vi "Set PressureDisplay Setup.vi"(8 "error in (no error)":errorcluster, 10 "PressureDisplay Setup":T1[](array[typedef]) {"Threshold" format="%#.1e"}, 11 "VacuumLines Configuration in":refnum<class "VacuumLines Configuration.lvclass">) -> (0 "error out":errorcluster, 3 "VacuumLines Configuration out":refnum<class "VacuumLines Configuration.lvclass">)   [LabVIEW 2016, in "Hardware.lvlib" / "VacuumLine.lvlib" / "VacuumLines Configuration.lvclass"]
uses:
  <userlib>/Common Components/Hardware/Abstract System/VacuumLine/VacuumLines Configuration/VacuumLines Configuration.lvclass
  <userlib>/Common Components/Hardware/Abstract System/VacuumLine/VacuumLines/Gauge Param.ctl
  <userlib>/Common Components/Hardware/Abstract System/VacuumLine/VacuumLines Configuration/VacuumLines Configuration.lvclass/VacuumLines Configuration.ctl
  <userlib>/Common Components/Hardware/Abstract System/VacuumLine/VacuumLines/VacuumLines.lvclass/VacuumLines.ctl
  <userlib>/Common Components/Hardware/Abstract System/VacuumLine/VacuumLines/VacuumLines.lvclass
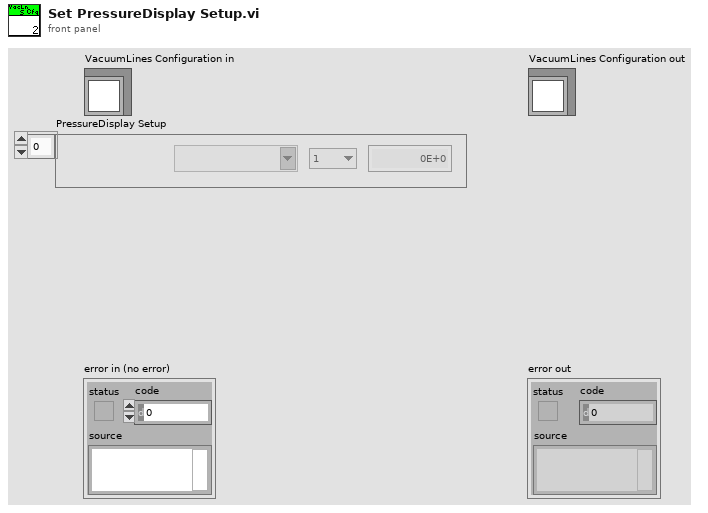
[diagram p1: front panel]
types:
  T1 = typedef "Hardware.lvlib/VacuumLine.lvlib/VacuumLines.lvclass/Gauge Param.ctl" = cluster{"label":string, "Gauge Controller":string, "Channel":enum16{"1", "2", "3", "4", "5", "6", "7", "8"}, "Threshold":dbl}
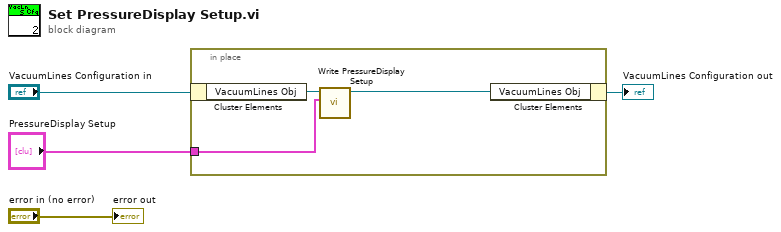
[diagram p0: block diagram]
diagram:
  n1 = in-place {
    in-place-border: "PressureDisplay Setup" -> [w5]
    n2 = in-place-cluster #1("VacuumLines Configuration in") -> ("VacuumLines Obj"=w7:refnum<class "VacuumLines.lvclass">)
    n3 = call <userlib>:"Write PressureDisplay Setup.vi"("PressureDisplay Setup"=w5, "VacuumLines in"=w7) -> ("VacuumLines out"=w6:refnum<class "VacuumLines.lvclass">)  [unwired: 9 in]
    n4 = in-place-cluster #1("VacuumLines Obj"=w6) -> (→"VacuumLines Configuration out":refnum<class "VacuumLines Configuration.lvclass">)
  }
  "error out" <- "error in (no error)"
